vi "getValue.vi"(8 "error in (no error)":errorcluster, 11 "Enumeration in":refnum<class "IEnumeration.lvclass">) -> (0 "error out":errorcluster, 2 "Value out":string, 3 "Enumeration out":refnum<class "IEnumeration.lvclass">)   [LabVIEW 2022 SP3, in "openDAQ.lvlib" / "daqCoreTypes.lvlib" / "IEnumeration.lvclass"]
uses:
  <instrlib>/openDAQ/Public/Classes/daqCoreTypes/IEnumeration/IEnumeration.lvclass
  C:/Program Files (x86)/National Instruments/LabVIEW 2022/instr.lib/openDAQ/Public/Classes/IBaseObject/IBaseObject.lvclass
  <instrlib>/openDAQ/Public/Classes/IBaseObject/IBaseObject.lvclass/IBaseObject.ctl
  <instrlib>/openDAQ/Public/Classes/IBaseObject/Accessor/Write reference.vi
  <instrlib>/openDAQ/Public/Classes/IBaseObject/Accessor/Read reference.vi
  <instrlib>/openDAQ/Public/Classes/daqCoreTypes/IString/IString.lvclass
  <instrlib>/openDAQ/Binaries/Windows/x86/copendaq32.dll
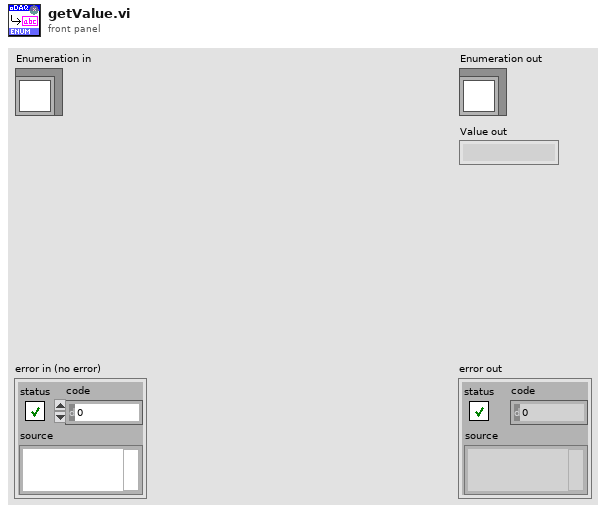
[diagram p1: front panel]
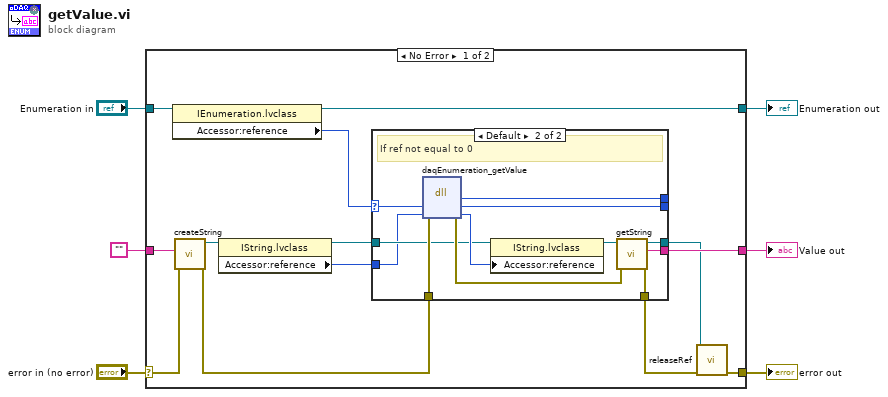
[diagram p0: block diagram]
diagram:
  n1 = case shown="No Error" "error in (no error)" {
    selector: "error in (no error)" -> [w12 w35]
    tunnel: [w16 w35] -> w5
    tunnel: [w17 w34] -> w3
    tunnel: "Enumeration in" -> [w19 w34]
    tunnel: [w15 _] -> w2
    tunnel: "" -> [w10 _]
    frame No Error {
      n2 = property class="IEnumeration.lvclass"(reference=w19) -> (reference out=w17:refnum<class "IEnumeration.lvclass">, "Accessor:reference"=w18:i64)  [unwired: 1 in, 1 out]
      n3 = call <instrlib>:"createString.vi"("error in (no error)"=w12, "String"=w10) -> ("error out"=w11:errorcluster, "IString out"=w9:refnum<class "IString.lvclass">)  [unwired: 8 in]
      n4 = property class="IString.lvclass"(reference=w9) -> (reference out=w8:refnum<class "IString.lvclass">, "Accessor:reference"=w7:i64)  [unwired: 1 in, 1 out]
      n5 = case shown="Default" w18 {
        selector: w18 -> [_ w31]
        tunnel: w11 -> [w20 w32]
        tunnel: [_ w29] -> w15
        tunnel: w8 -> [w21 w25]
        tunnel: [w21 w28] -> w14
        tunnel: [w20 w26] -> w13
        tunnel: [_ w24] -> _
        tunnel: w7 -> [_ w22]
        tunnel: [_ w23] -> _
        frame 0 {
        }
        frame Default {
          # "If ref not equal to 0"
          n6 = dll-call lib="C:/Program Files (x86)/National Instruments/LabVIEW 2022/instr.lib/openDAQ/Binaries/Windows/x86/copendaq*.*" fn="daqEnumeration_getValue"(error in=w32, "enum"=w31, "value"=w22) -> (error out=w27:errorcluster, "return type"=w24:u32, "enum"=w23:i64, "value"=w33:i64)  [unwired: 2 in, 1 out]
          n7 = property class="IString.lvclass"(reference=w25, "Accessor:reference"=w33) -> (reference out=w30:refnum<class "IString.lvclass">)  [unwired: 1 in, 1 out]
          n8 = call <instrlib>:"getString.vi"("error in (no error)"=w27, "IString in"=w30) -> ("error out"=w26:errorcluster, "String out"=w29:string, "IString out"=w28:refnum<class "IString.lvclass">)  [unwired: 7 in]
        }
      }
      n9 = call-dynamic "releaseRef.vi"("error in (no error)"=w13, "IBaseObject in"=w14) -> ("error out"=w16:errorcluster)  [unwired: 9 in]
    }
    frame Error {
    }
  }
  "error out" <- w5
  "Enumeration out" <- w3
  "Value out" <- w2
